vi "PDO Mapping.vi"(8 "error in":errorcluster, 9 "PDO Mapping T":string(combo)="Transmit PDO mapping 1", 10 "PDO Mapping R":string(combo)="Receive PDO mapping 1", 11 "ro/r/w":T1=enum."Read Only") -> (0 "error out":errorcluster, 2 "PDO Mapping":string, 3 "ro/r/w":T1=enum."Read Only")   [LabVIEW 2016, in "Motor Base.lvlib" / "Motor Base.lvclass"]
uses:
  Motor Base.lvclass
  AccessType.ctl
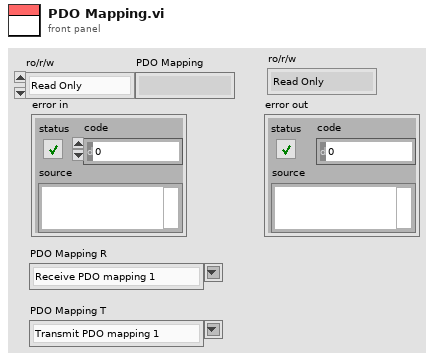
[diagram p1: front panel]
types:
  T1 = typedef "Motor Base.lvlib/Motor Base.lvclass/AccessType.ctl" = enum16{"Write", "Read", "Read Only"}
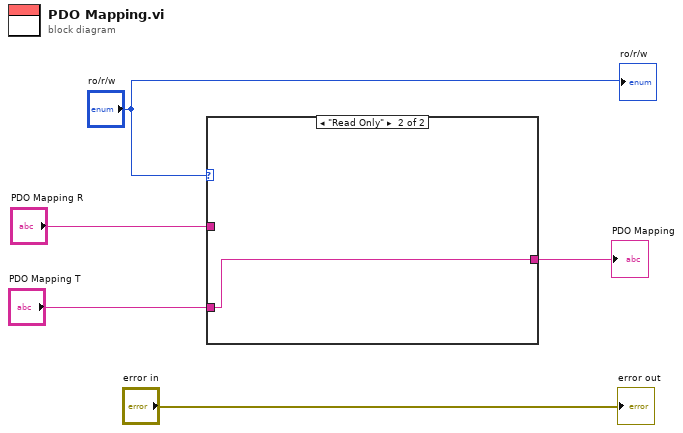
[diagram p0: block diagram]
diagram:
  n1 = case shown="\"Read Only\"" "ro/r/w" {
    tunnel: [w6 w7] -> w5
    tunnel: "PDO Mapping R" -> [w6 _]
    tunnel: "PDO Mapping T" -> [_ w7]
    frame "Write", "Read", Default {
    }
    frame "Read Only" {
      # "默认都是使用mapping 1"
    }
  }
  "PDO Mapping" <- w5
  "error out" <- "error in"
  "ro/r/w" <- "ro/r/w"
